vi "ma_Locate three fingers (amplitude input).vi"(2 "spectrum includes end points?":bool, 3 "criterion":T2 {"Threshold" format="%.2f"}, 4 "spectral info":T1 {"window" items=["Rectangle"=0, "Hanning"=1, "Hamming"=2, "Blackman-Harris"=3, "Exact Blackman"=4, "Blackman"=5, "Flat Top"=6, "4 Term B-Harris "=7, "7 Term B-Harris"=8, "Low Sidelobe"=9, "Blackman Nuttall"=11, "Triangle"=30, "Bartlett-Hanning"=31, "Bohman"=32, "Parzen"=33, "Welch"=34, "Kaiser"=60, "Dolph-Chebyshev"=61, "Gaussian"=62]}, 5 "FFT spectrum":T3={"f0"=0.0, "df"=1.0, "spectrum"=[]} {"spectrum" format="%.2f"; "df" format="%.2f"; "f0" format="%.2f"}) -> (0 "number of tones":i32, 1 "three fingers (frequency normalized)":T3[](array[typedef]) {"spectrum" format="%.2f"; "df" format="%.2f"; "f0" format="%.2f"})   [LabVIEW 2020, in "NI_MAPro.lvlib"]
uses:
  NI_MAPro.lvlib
  ma_sml_Spectrum Cluster (real).ctl
  ma_sml_Spectral Info.ctl
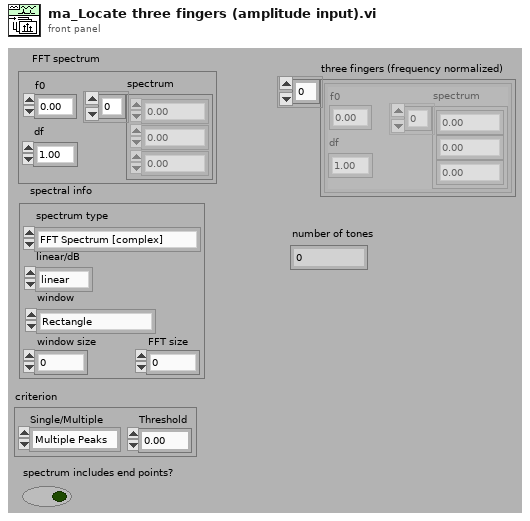
[diagram p1: front panel]
types:
  T1 = typedef "NI_MAPro.lvlib/ma_sml_Spectral Info.ctl" = cluster{"spectrum type":enum16{"FFT Spectrum [complex]", "Amplitude [Magnitude]", "Power [Magnitude^2]", "Cross Spectrum [complex]", "Frequency Response [Complex]"}, "linear/dB":enum16{"linear", "dB"}, "window":u16, "window size":i32, "FFT size":i32}
  T2 = cluster{"Single/Multiple":enum16{"Multiple Peaks", "Single Max Peak"}, "Threshold":dbl}
  T3 = typedef "NI_MAPro.lvlib/ma_sml_Spectrum Cluster (real).ctl" = cluster{"f0":dbl, "df":dbl, "spectrum":dbl[]}
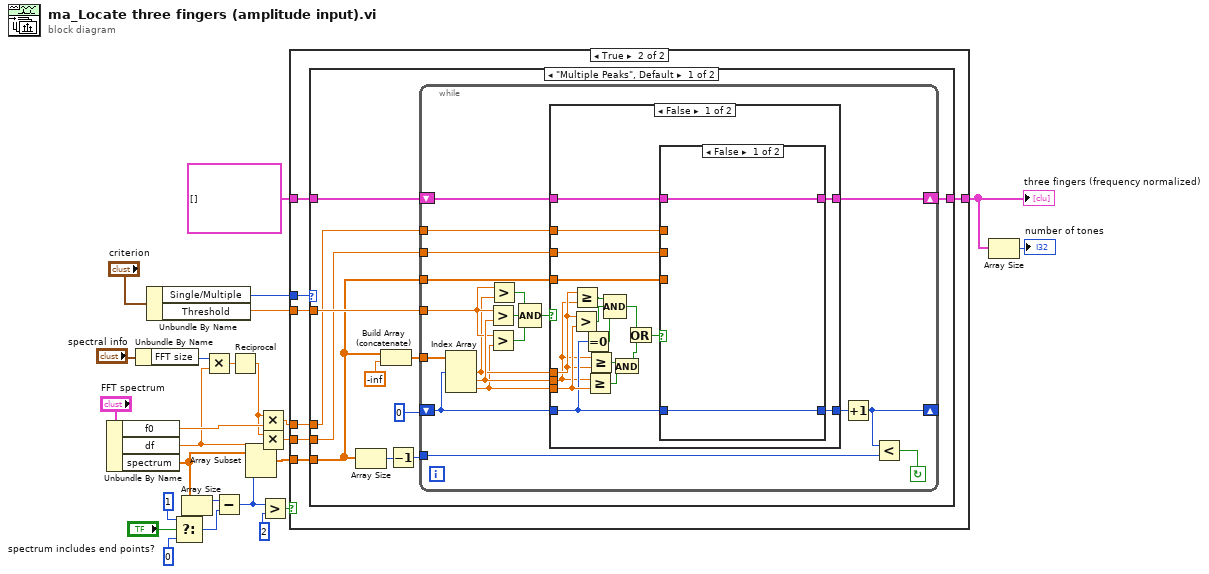
[diagram p0: block diagram]
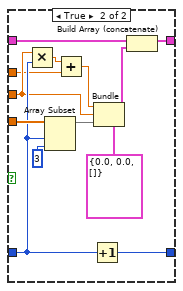
[diagram p3: hidden frame]
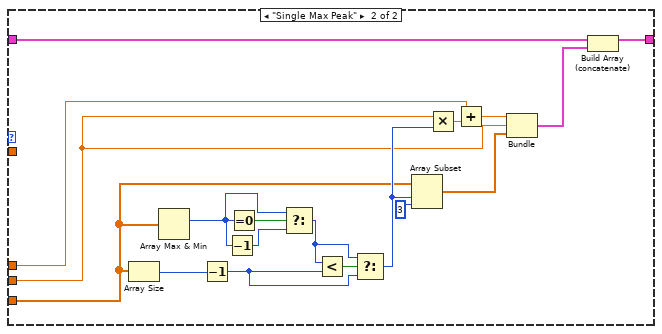
[diagram p5: hidden frame]
diagram:
  n1 = Unbundle By Name("FFT spectrum") -> ("f0"=w15:dbl, "df"=w12:dbl, "spectrum"=w3:dbl[])
  n2 = Unbundle By Name("spectral info") -> ("FFT size"=w13:i32)
  n3 = Unbundle By Name("criterion") -> ("Single/Multiple"=w20:enum16{"Multiple Peaks", "Single Max Peak"}, "Threshold"=w21:dbl)
  n4 = Select(t=1, s="spectrum includes end points?", f=0) -> (s? t:f=w8:i32)
  n5 = Array Size(array=w3) -> (size(s)=w9:i32)
  n6 = Multiply(x=w13, y=w12) -> (x*y=w11:dbl)
  n7 = Subtract(x=w9, y=w8) -> (x-y=w2:i32)
  n8 = Reciprocal(x=w11) -> (1/x=w10:dbl)
  n9 = Array Subset(array=w3, length=w2) -> (w4:dbl[])  [unwired: 1 in]
  n10 = Multiply(x=w10, y=w15) -> (x*y=w17:dbl)
  n11 = Multiply(x=w10, y=w12) -> (x*y=w16:dbl)
  n12 = Greater?(x=w2, y=2) -> (0:w24:bool)
  n13 = case shown="True" w24 {
    tunnel: w21 -> [_ w33]
    tunnel: w17 -> [_ w32]
    tunnel: w16 -> [_ w31]
    tunnel: [w26 w30] -> w19
    tunnel: w4 -> [_ w29]
    tunnel: T3[] [] ("three fingers (frequency normalized)") -> [w26 w28]
    tunnel: w20 -> [_ w27]
    frame False {
    }
    frame True {
      n14 = case shown="\"Multiple Peaks\", Default" w27 {
        tunnel: w33 -> [w41 _]
        tunnel: w32 -> [w40 w106]
        tunnel: w31 -> [w39 w104]
        tunnel: [w38 w100] -> w30
        tunnel: w29 -> [w34 w99]
        tunnel: w28 -> [w35 w102]
        frame "Multiple Peaks", Default {
          n15 = Array Size(array=w34) -> (size(s)=w37:i32)
          n16 = Build Array (concatenate)(w34, -inf ("df")) -> (w43:dbl[])
          n17 = Decrement(x=w37) -> (x-1=w36:i32)
          n18 = while {
            tunnel: w36 -> [w52]
            tunnel: w39 -> [w56]
            tunnel: w40 -> [w57]
            tunnel: w34 -> [w58]
            shift-left: w35 -> [w59]
            shift-right: [w55] -> w38
            tunnel: w41 -> [w50]
            shift-left: 0 -> [w61]
            shift-right: [w53] -> _
            tunnel: w43 -> [w63]
            stop <- w54 continue-if-true
            n19 = Index Array(array=w63, index #1=w61) -> (element #1=w49:dbl, element #2=w51:dbl, element #3=w48:dbl)  [unwired: 2 in]
            n20 = Greater?(x=w50, y=w51) -> (0:w62:bool)
            n21 = Greater?(x=w50, y=w48) -> (0:w45:bool)
            n22 = Greater?(x=w50, y=w49) -> (0:w46:bool)
            n23 = Compound Arithmetic op=AND(w46, w62, w45) -> (w47:bool)
            n24 = case shown="False" w47 {
              tunnel: [w79 w98] -> w60
              tunnel: w61 -> [w69 w98]
              tunnel: w48 -> [w73 _]
              tunnel: w49 -> [w65 _]
              tunnel: w59 -> [w78 w97]
              tunnel: w58 -> [w77 _]
              tunnel: w57 -> [w76 _]
              tunnel: w56 -> [w75 _]
              tunnel: [w74 w97] -> w55
              tunnel: w51 -> [w64 _]
              frame False {
                n25 = Greater?(x=w65, y=w73) -> (0:w71:bool)
                n26 = Greater Or Equal?(x=w65, y=w64) -> (x >= y?=w72:bool)
                n27 = Equal To 0?(x=w69) -> (x = 0?=w70:bool)
                n28 = Greater Or Equal?(x=w64, y=w73) -> (x >= y?=w80:bool)
                n29 = Greater Or Equal?(x=w64, y=w65) -> (x >= y?=w81:bool)
                n30 = Compound Arithmetic op=AND(w72, w71, w70) -> (w66:bool)
                n31 = And(x=w81, y=w80) -> (x .and. y?=w68:bool)
                n32 = Or(x=w66, y=w68) -> (x .or. y?=w67:bool)
                n33 = case shown="False" w67 {
                  tunnel: w69 -> [w83 w94]
                  tunnel: [w83 w96] -> w79
                  tunnel: w78 -> [w82 w87]
                  tunnel: w77 -> [_ w95]
                  tunnel: w76 -> [_ w89]
                  tunnel: w75 -> [_ w91]
                  tunnel: [w82 w85] -> w74
                  frame False {
                  }
                  frame True {
                    n34 = Multiply(x=w91, y=w94) -> (x*y=w90:dbl)
                    n35 = Array Subset(array=w95, index=w94, length=3 ("Array Length")) -> (w92:dbl[])
                    n36 = Add(x=w90, y=w89) -> (x+y=w88:dbl)
                    n37 = Increment(x=w94) -> (x+1=w96:i32)
                    n38 = Bundle(cluster=T3 {"f0"=0.0, "df"=0.0, "spectrum"=[]} ("FFT spectrum"), "f0"=w88, "df"=w91, "spectrum"=w92) -> (w86:T3)
                    n39 = Build Array (concatenate)(w87, w86) -> (w85:T3[])
                  }
                }
              }
              frame True {
              }
            }
            n40 = Increment(x=w60) -> (x+1=w53:i32)
            n41 = Less?(x=w53, y=w52) -> (x < y?=w54:bool)
          }
        }
        frame "Single Max Peak" {
          n42 = Array Size(array=w99) -> (size(s)=w108:i32)
          n43 = Array Max & Min(array=w99) -> (max index (indices)=w112:i32)  [unwired: 3 out]
          n44 = Decrement(x=w108) -> (x-1=w107:i32)
          n45 = Decrement(x=w112) -> (x-1=w113:i32)
          n46 = Equal To 0?(x=w112) -> (x = 0?=w114:bool)
          n47 = Select(t=w112, s=w114, f=w113) -> (s? t:f=w110:i32)
          n48 = Less?(x=w110, y=w107) -> (x < y?=w111:bool)
          n49 = Select(t=w110, s=w111, f=w107) -> (s? t:f=w109:i32)
          n50 = Array Subset(array=w99, index=w109, length=3 ("Array Length")) -> (w103:dbl[])
          n51 = Multiply(x=w104, y=w109) -> (x*y=w115:dbl)
          n52 = Add(x=w106, y=w115) -> (x+y=w105:dbl)
          n53 = Bundle(w105, w104, w103) -> (w101:cluster{dbl, dbl, dbl[]})  [unwired: 1 out]
          n54 = Build Array (concatenate)(w102, w101) -> (w100:T3[])
        }
      }
    }
  }
  "three fingers (frequency normalized)" <- w19
  n55 = Array Size(array=w19) -> (size(s)=→"number of tones":i32)
